vi "Write Publish Msg.vi"(10 "Pre-Addressed Publish Msg":refnum<class "Publish Msg.lvclass">, 11 "IModel in":refnum<class "IModel.lvclass">) -> (3 "IModel out":refnum<class "IModel.lvclass">)   [LabVIEW 2015, in "IModel.lvlib" / "IModel.lvclass"]
uses:
  IModel.lvclass
  IMediator/IMediator Messages/Publish Msg/Publish Msg.lvclass
  IModel.lvclass/IModel.ctl
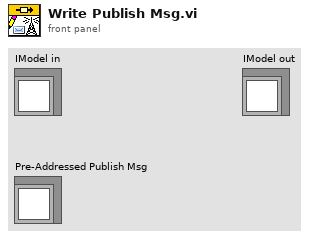
[diagram p1: front panel]
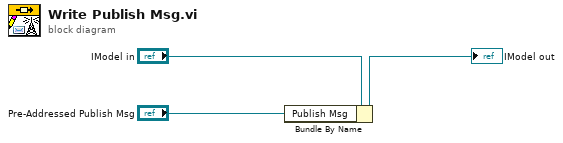
[diagram p0: block diagram]
diagram:
  n1 = Bundle By Name(cluster="IModel in", "Publish Msg"="Pre-Addressed Publish Msg") -> (→"IModel out":refnum<class "IModel.lvclass">)
